vi "Read Mac Address.vi"(8 "error in (no error)":errorcluster, 11 "TrialBasedExperiment in":refnum<class "MatlabExperiment.lvclass">) -> (0 "error out":errorcluster, 2 "Mac Address":string, 3 "TrialBasedExperiment out":refnum<class "MatlabExperiment.lvclass">)   [LabVIEW 2011, in "MatlabExperiment.lvclass"]
uses:
  MatlabExperiment.lvclass
  MatlabExperiment.lvclass/MatlabExperiment.ctl
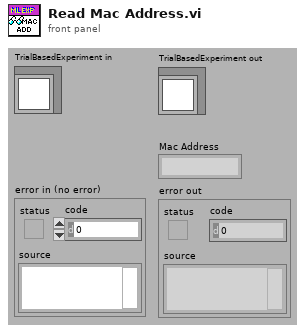
[diagram p1: front panel]
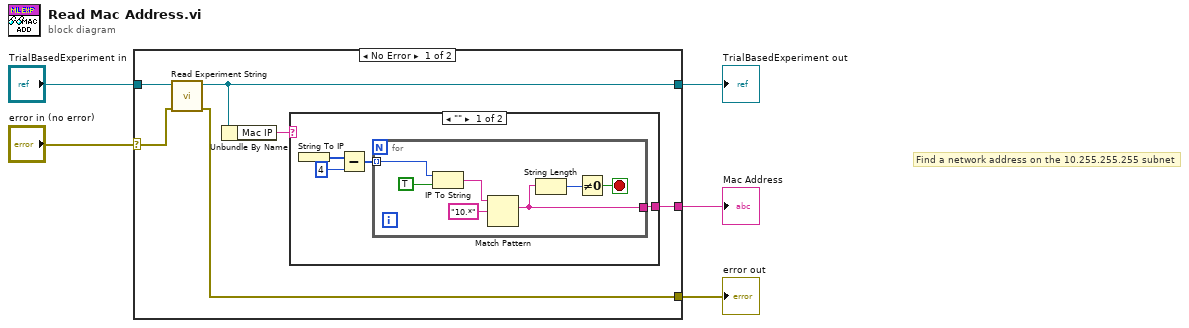
[diagram p0: block diagram]
diagram:
  # "Find a network address on the 10.255.255.255 subnet"
  n1 = case shown="No Error" "error in (no error)" {
    selector: "error in (no error)" -> [w9 w24]
    tunnel: [w8 w24] -> w4
    tunnel: [w7 w25] -> w2
    tunnel: "TrialBasedExperiment in" -> [w10 w25]
    tunnel: [w11 _] -> w1
    frame No Error {
      n2 = call-dynamic "Read Experiment String.vi"("error in (no error)"=w9, "TrialBasedExperiment in"=w10) -> ("error out"=w8:errorcluster, "TrialBasedExperiment out"=w7:refnum<class "MatlabExperiment.lvclass">)  [unwired: 7 in, 1 out]
      n3 = Unbundle By Name(w7) -> ("Mac IP"=w6:string)
      n4 = case shown="\"\"" w6 {
        selector: w6 -> [_ w23]
        tunnel: [w12 w23] -> w11
        frame "" {
          n5 = String To IP() -> (0:w13:u32[])  [unwired: 1 out]
          n6 = Subtract(x=w13, y=u32 4) -> (x-y=w15:u32[])
          n7 = for {
            tunnel: w15 -> [w21] mode=indexing
            tunnel: [w18] -> w12
            stop <- w16 stop-if-true
            n8 = IP To String(1:TRUE ("dot notation? (F)"), 2:w21) -> (0:w20:string)
            n9 = Match Pattern(string=w20, regular expression="10.*") -> (match substring=w18:string)  [unwired: 1 in, 3 out]
            n10 = String Length(string=w18) -> (length=w17:i32)
            n11 = Not Equal To 0?(x=w17) -> (x != 0?=w16:bool)
          }
        }
        frame "1", Default {
        }
      }
    }
    frame Error {
    }
  }
  "error out" <- w4
  "TrialBasedExperiment out" <- w2
  "Mac Address" <- w1
